vi "Range.vi"(6 "y":i32, 7 "x":i32) -> (1 "Range":i32[](array[numeric]))   [LabVIEW 2019]
doc: "Given x, y, return a 1D array of incrementing values in [min(x,y), max(x,y)]."
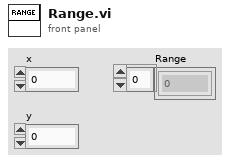
[diagram p1: front panel]
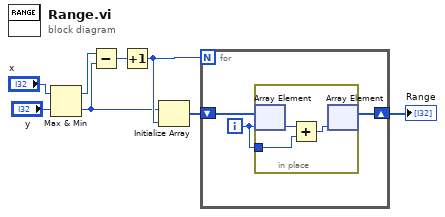
[diagram p0: block diagram]
diagram:
  n1 = Max & Min(x="x", y="y") -> (max(x,y)=w3:i32, min(x,y)=w4:i32)
  n2 = Subtract(x=w3, y=w4) -> (x-y=w7:i32)
  n3 = Increment(x=w7) -> (x+1=w8:i32)
  n4 = Initialize Array(w4, w8) -> (w5:i32[])
  n5 = for {
    N: w8 -> [_]
    shift-right: [w9] -> w6
    shift-left: w5 -> [w11]
    i -> [w10]
    n6 = in-place {
      in-place-border: w10 -> [w14]
      n7 = in-place-array #1(w11, w10) -> (w13:i32)
      n8 = Add(x=w13, y=w14) -> (x+y=w12:i32)
      n9 = in-place-array #1(w12) -> (w9:i32[])  [unwired: 1 out]
    }
  }
  "Range" <- w6
